vi "Pre Launch Init.vi"(11 "Mediator in":refnum<class "BusMediator.lvclass">) -> (0 "error out":errorcluster, 3 "Mediator out":refnum<class "BusMediator.lvclass">)   [LabVIEW 2017, in "BusMediator.lvclass"]
doc: "(<B>Filename</B>: Actor Framework.lvlib:Actor.lvclass:Pre Launch Init.vi)\n\nDefines behavior that occurs after the Launch Nested Actor method is invoked but before the actor's Actor Core method begins running.\n\nBy default, this method does nothing. A descendant class may override it to define behavior."
uses:
  BusMediator.lvclass
  <vilib>/Composed/GPM Packages/mva-framework/Source/Framework/IMediator/IMediator/IMediator.lvclass
  TopicLookupTable/TopicLookupTable.lvclass
  <vilib>/Composed/GPM Packages/mva-framework/Source/Framework/IMediator/IMediator Messages/Start Bus Monitor Msg/Start Bus Monitor Msg.lvclass
  <vilib>/ActorFramework/Actor/Actor.lvclass
  C:/Program Files (x86)/National Instruments/LabVIEW 2017/vi.lib/Composed/GPM Packages/mva-framework/Source/Framework/IMediator/IMediator/IMediator.lvclass
  C:/Program Files (x86)/National Instruments/LabVIEW 2017/vi.lib/ActorFramework/Actor/Actor.lvclass
  <vilib>/ActorFramework/Message Enqueuer/Message Priority.ctl
  <vilib>/ActorFramework/Message Enqueuer/Message Enqueuer.lvclass
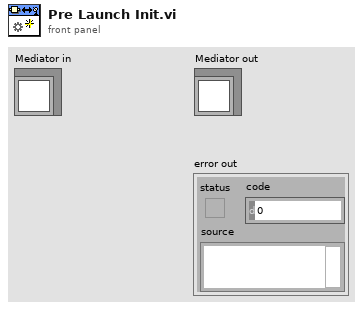
[diagram p1: front panel]
types:
  T1 = typedef "Actor Framework.lvlib/Message Enqueuer.lvclass/Message Priority.ctl" = enum16{"Low", "Normal", "High"}
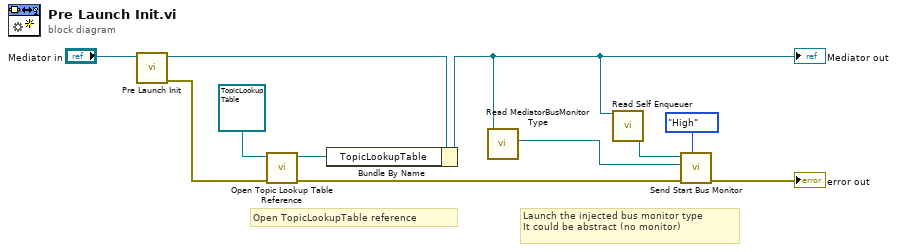
[diagram p0: block diagram]
diagram:
  # "Launch the injected bus monitor type\nIt could be abstract (no monitor)"
  # "Open TopicLookupTable reference"
  n1 = call-parent "Pre Launch Init.vi"("IMediator In"="Mediator in") -> ("error out"=w8:errorcluster, "IMediator Out"=w11:refnum<class "BusMediator.lvclass">)  [unwired: 9 in]
  n2 = call "Open Topic Lookup Table Reference.vi"("error in (no error)"=w8, "TopicLookupTable in"=refnum<class "TopicLookupTable.lvclass"> refnum ("Mediator.lvlib:TopicLookupTable.lvclass")) -> ("error out"=w7:errorcluster, "TopicLookupTable Reference"=w9:refnum<data-value>)  [unwired: 8 in]
  n3 = Bundle By Name(cluster=w11, "TopicLookupTable"=w9) -> (w3:refnum<class "BusMediator.lvclass">)
  "Mediator out" <- w3
  n4 = call <vilib>:"Read MediatorBusMonitor Type.vi"("IMediator in"=w3) -> ("MediatorBusMonitor (Type)"=w4:refnum<class "IMediatorBusMonitor.lvclass">)  [unwired: 10 in]
  n5 = call <vilib>:"Read Self Enqueuer.vi"("Actor"=w3) -> ("Self Enqueuer"=w2:refnum<class "Message Enqueuer.lvclass">)  [unwired: 10 in]
  n6 = call <vilib>:"Send Start Bus Monitor.vi"("Message Priority (Normal)"=Message_Priority."High", "error in (no error)"=w7, "MediatorBusMonitor (Type)"=w4, "Message Enqueuer"=w2) -> ("error out"=→"error out":errorcluster)  [unwired: 6 in, 1 out]
